vi "Distance to horizontal distance.vi"(1 "Camera High (ft) (constant)":dbl, 3 "Distance (ft)":dbl) -> (0 "Horizontal Distance (ft)":dbl)   [LabVIEW 2013]
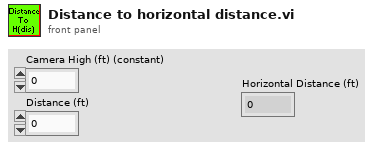
[diagram p1: front panel]
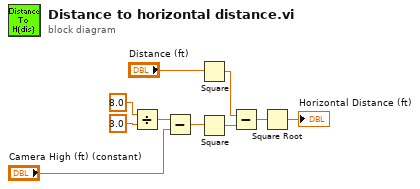
[diagram p0: block diagram]
diagram:
  n1 = Divide(x=8.0, y=3.0) -> (x/y=w1:dbl)
  n2 = Subtract(x=w1, y="Camera High (ft) (constant)") -> (x-y=w6:dbl)
  n3 = Square(x="Distance (ft)") -> (x^2=w10:dbl)
  n4 = Square(x=w6) -> (x^2=w9:dbl)
  n5 = Subtract(x=w10, y=w9) -> (x-y=w8:dbl)
  n6 = Square Root(x=w8) -> (sqrt(x)=→"Horizontal Distance (ft)":dbl)
